vi "Main.vi"() -> ()   [LabVIEW 2020]
panel:
  out "Loading":u8(slide) scale=0.0..100.0
  out "Load Time (s)":dbl
  out "Enties":i32
  out "Header String":string
  out "Valid?":bool
  out "Version":string
  in  "File Path":path
  out "Entity Tree":string(tree)
  in  "Tab Control":enum32{"Graph", "Strings"}(tab)
  out "XY Graph":cluster{"X":dbl, "Y":dbl}[](graph)
  in  "Pause":bool
  in  "Start":bool
  in  "NT Time":dbl(slide) scale=0.0..10.0
  in  "Start NT":bool
  # "DataLog Viewer"
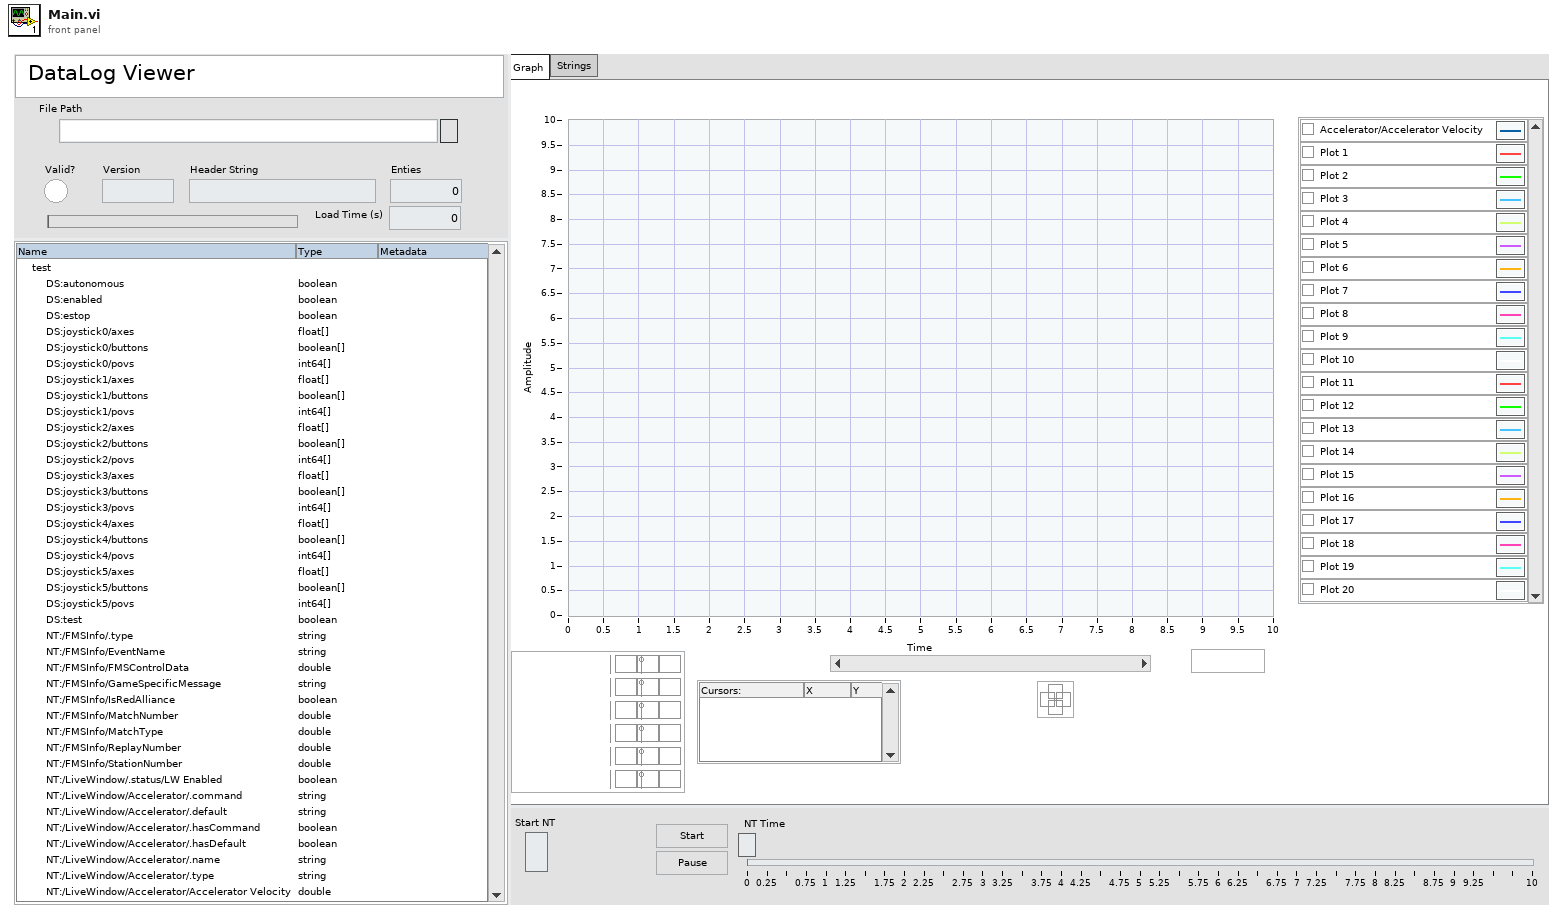
[diagram p1: front panel]
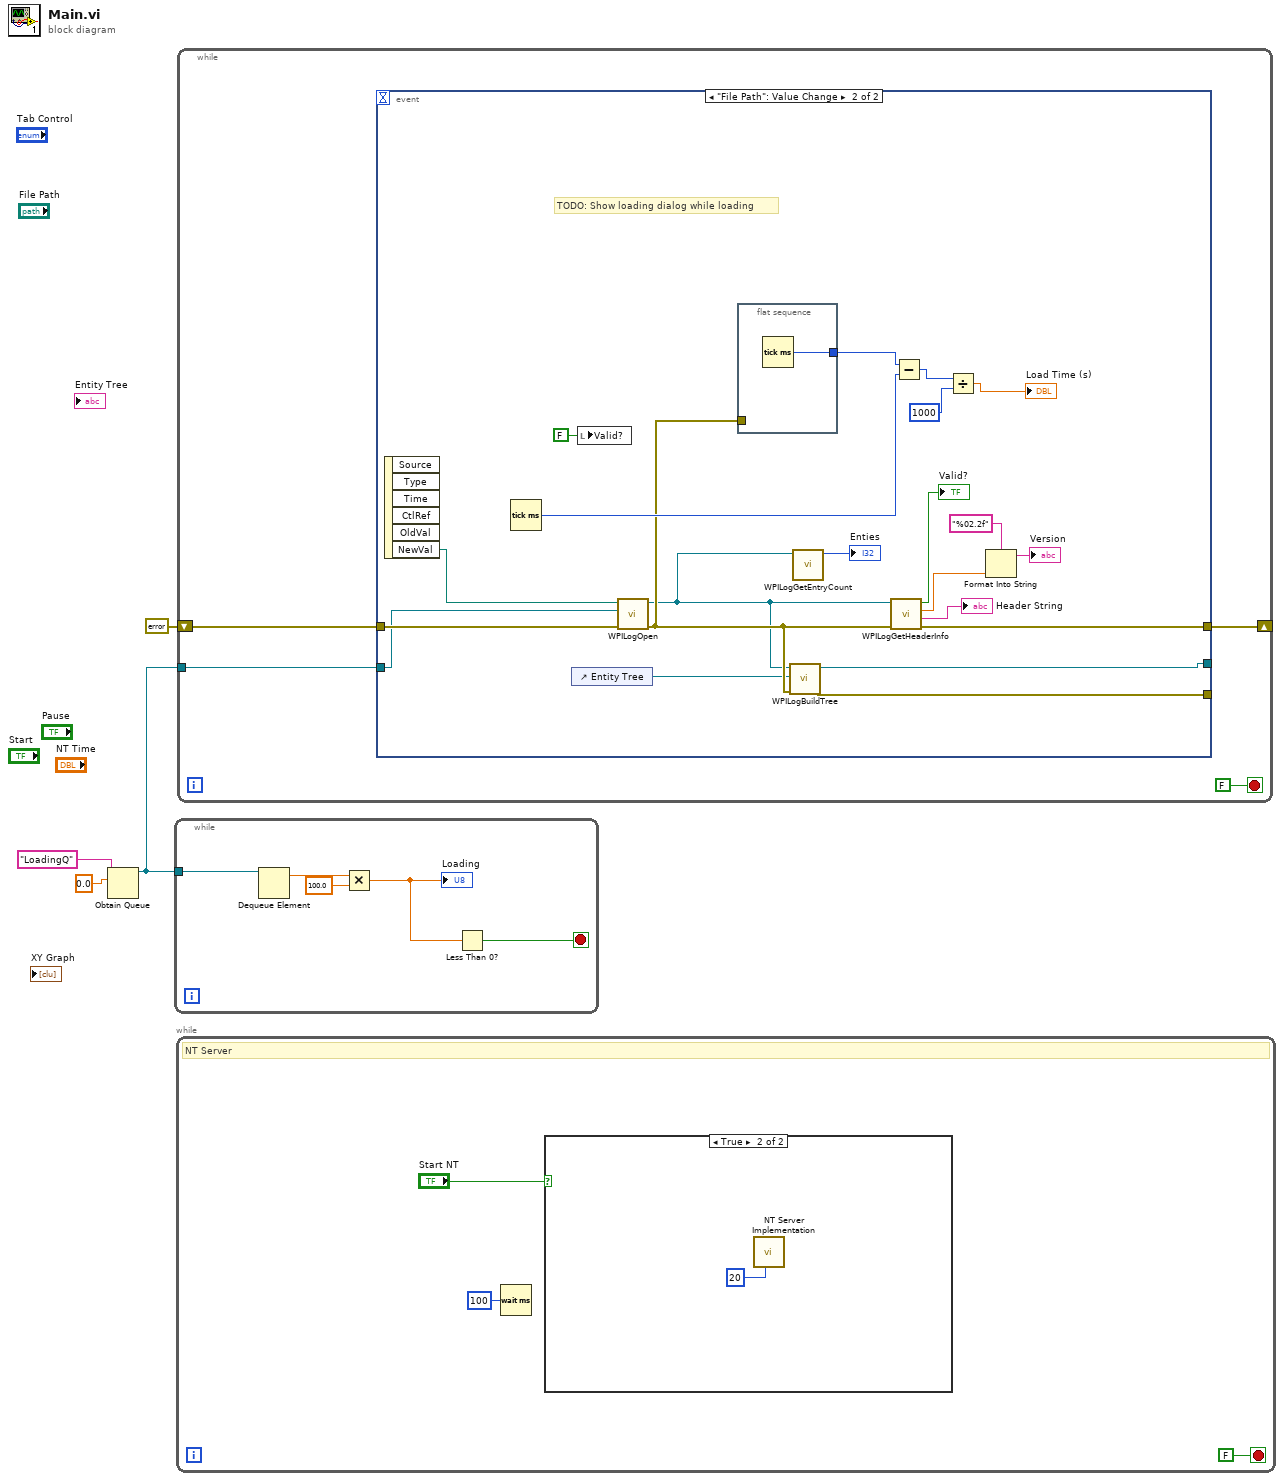
[diagram p0: block diagram]
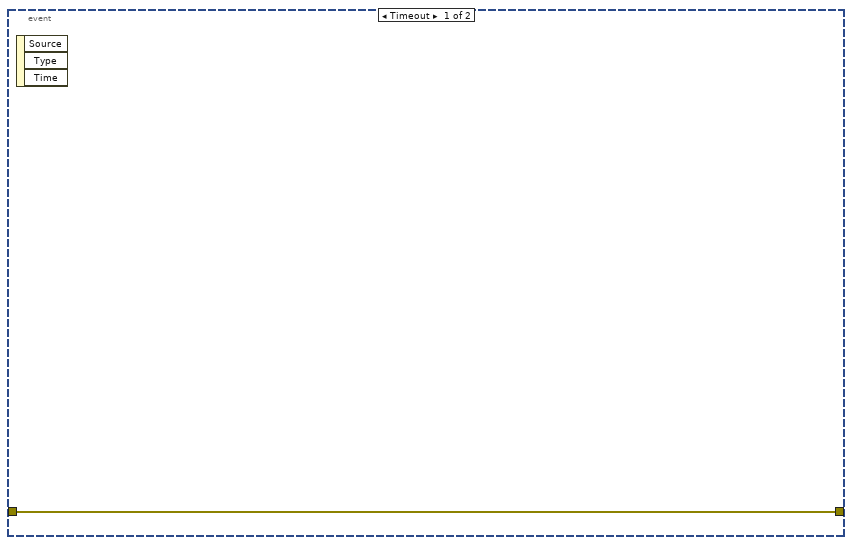
[diagram p3: hidden frame]
diagram:
  n1 = Obtain Queue(name (unnamed)="LoadingQ", element data type=0.0) -> (queue out=w1:refnum<queue>)  [unwired: 3 in, 2 out]
  n2 = while {
    tunnel: w1 -> [w9]
    stop <- w5 stop-if-true
    n3 = Dequeue Element(queue=w9) -> (element=w8:dbl)  [unwired: 2 in, 3 out]
    n4 = Multiply(x=w8, y=100.0) -> (x*y=w6:dbl)
    "Loading" <- w6
    n5 = Less Than 0?(x=w6) -> (x < 0?=w5:bool)
  }
  n6 = while {
    stop <- FALSE stop-if-true
    # "NT Server"
    n7 = Wait (ms)(milliseconds to wait=u32 100) -> ()  [unwired: 1 out]
    n8 = case shown="True" "Start NT" {
      frame False {
      }
      frame True {
        n9 = call <vilib>:"NT Server Implementation.vi"("Update Time"=20) -> ()  [unwired: 11 in]
      }
    }
  }
  n10 = while {
    shift-right: [w16] -> _
    shift-left: errorcluster {"status"=FALSE, "code"=0, "source"=""} ("error out") -> [w15]
    tunnel: w1 -> [w14]
    stop <- FALSE stop-if-true
    n11 = event shown="[1] \"File Path\": Value Change" {
      selector: _ -> [_ _]
      dyn-events: _ -> [_ _]
      timeout: _ -> [_ _]
      tunnel: [w18 w33] -> w16
      tunnel: w15 -> [w18 w39]
      tunnel: w14 -> [_ w24]
      tunnel: [_ w21] -> _
      tunnel: [_ w20] -> _
      event Timeout {
        n12 = event-data() -> ()  [unwired: 1 in, 3 out]
      }
      event "File Path": Value Change {
        # "TODO: Show loading dialog while loading"
        n13 = event-data() -> ("NewVal"=w38:path)  [unwired: 1 in, 5 out]
        n14 = Tick Count (ms)() -> (millisecond timer value=w29:u32)
        n15 = control-ref of="Entity Tree"() -> (w22:refnum<vi>)
        n16 = local write "Valid?"(FALSE ("Valid?")) -> ()
        n17 = call "WPILogOpen.vi"("error in (no error)"=w39, "loading q"=w24, "File Path"=w38) -> ("error out"=w23:errorcluster, "WPILog Ref"=w19:refnum<data-value>)  [unwired: 7 in]
        n18 = flat-sequence {
          tunnel: w23 -> [_]
          tunnel: [w40] -> w30
          frame #0 {
            n19 = Tick Count (ms)() -> (millisecond timer value=w40:u32)
          }
        }
        n20 = call "WPILogBuildTree.vi"("error in (no error)"=w23, "Entity Tree"=w22, "Data Value Reference in"=w19) -> ("error out"=w21:errorcluster, "Data Value Reference out"=w20:refnum<data-value>)  [unwired: 7 in]
        n21 = call "WPILogGetEntryCount.vi"("Data Value Reference in"=w19) -> ("Entires"=→"Enties":i32)  [unwired: 9 in, 1 out]
        n22 = call "WPILogGetHeaderInfo.vi"("error in (no error)"=w23, "Data Value Reference in"=w19) -> ("error out"=w33:errorcluster, "Header Extra String"=→"Header String":string, "Version"=w36:dbl, "Boolean"=→"Valid?":bool)  [unwired: 6 in]
        n23 = Subtract(x=w30, y=w29) -> (x-y=w28:u32)
        n24 = Divide(x=w28, y=u32 1000) -> (x/y=→"Load Time (s)":dbl)
        n25 = Format Into String(format string="%02.2f", w36) -> (resulting string=→"Version":string)  [unwired: 2 in, 1 out]
      }
    }
  }
